vi "SlopeWrap.vi"(8 "Low Value":dbl, 9 "High Value":dbl, 10 "Low Angle":dbl, 11 "High Angle":dbl) -> (2 "0/360 Intercept":dbl, 3 "Slope":dbl)   [LabVIEW 2012]
doc: "Given the first inputted angle (0 or above 0) and the last inputted angle (highest angle less than 360) this will return the slope to attach to the last inputed angle and to attach to the 0/360 angle and also the intercept of the 0/360 point."
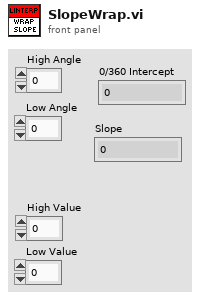
[diagram p1: front panel]
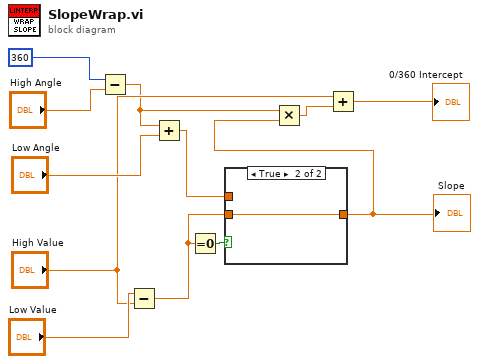
[diagram p0: block diagram]
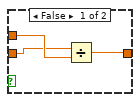
[diagram p2: hidden frame]
diagram:
  n1 = Subtract(x=360, y="High Angle") -> (x-y=w1:dbl)
  n2 = Subtract(x="Low Value", y="High Value") -> (x-y=w7:dbl)
  n3 = Add(x=w1, y="Low Angle") -> (x+y=w6:dbl)
  n4 = Equal To 0?(x=w7) -> (x = 0?=w8:bool)
  n5 = case shown="True" w8 {
    tunnel: w6 -> [w15 _]
    tunnel: w7 -> [w14 w16]
    tunnel: [w13 w16] -> w3
    frame False {
      n6 = Divide(x=w14, y=w15) -> (x/y=w13:dbl)
    }
    frame True {
    }
  }
  "Slope" <- w3
  n7 = Multiply(x=w1, y=w3) -> (x*y=w2:dbl)
  n8 = Add(x="High Value", y=w2) -> (x+y=→"0/360 Intercept":dbl)
